vi "Serial_Port_Packet_Read_Write_Test.vi"() -> ()   [LabVIEW 2017]
uses:
  Classes/ADCP.lvclass
panel:
  out "Packet frame ID":u8
  out "Packet node ID":u8
  out "Packet Type":T1(ring)
  out "Checksum Valid ?":bool
  out "Packet_Priority":enum16{"LOW", "HIGH"}(ring)
  out "Raw Packet Out":u8[](array[numeric])
  in  "Raw Packet In":u8[](array[numeric])
  in  "error in (no error)":errorcluster
  in  "Baud rate":u32
  in  "COM Port":refnum<visa-resource-name>
  in  "ADCP in":refnum<class "ADCP.lvclass">
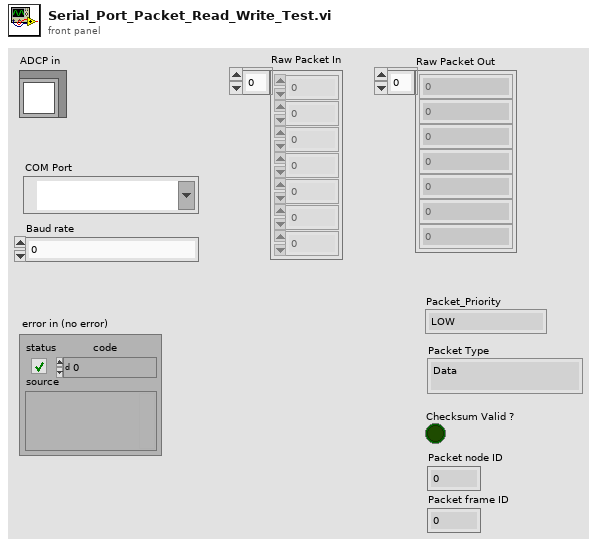
[diagram p1: front panel]
types:
  T1 = enum16{"Data", "Connection Management", "Remote Request", "Error and status", "INVALID"}
  T2 = cluster{"Symbol File Path":path, "Transmit Log File Path":path, "Receive Log File Path":path, "COM Port":refnum<visa-resource-name>, "Baud rate":u32, "Number of retries":u16, "Retry interval (ms)":u16, "Session start time (ms)":u32, "Current time (ms)":u32, "Serialport timeout (ms)":u32}
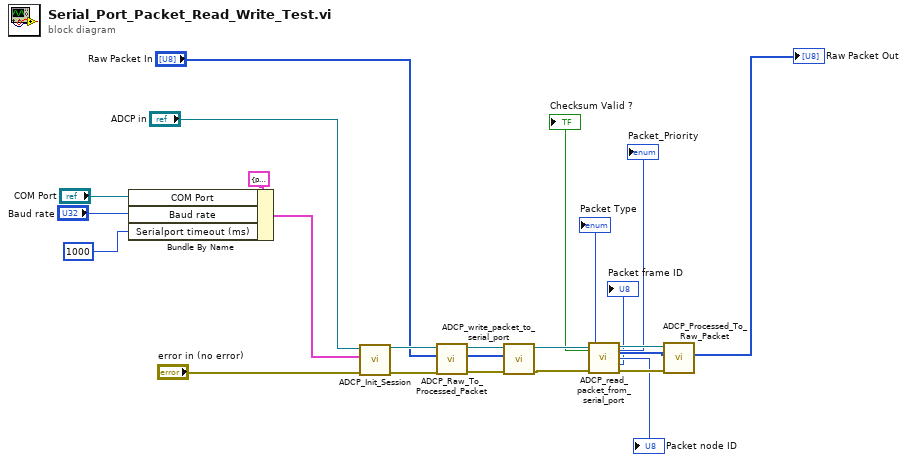
[diagram p0: block diagram]
diagram:
  n1 = Bundle By Name(cluster=T2 {"Symbol File Path"=path "", "Transmit Log File Path"=path "", "Receive Log File Path"=path "", "COM Port"="", "Baud rate"=0, "Number of retries"=0, "Retry interval (ms)"=0, "Session start time (ms)"=0, "Current time (ms)"=0, "Serialport timeout (ms)"=0} ("ADCP Session Parameters"), "COM Port"="COM Port", "Baud rate"="Baud rate", "Serialport timeout (ms)"=u32 1000) -> (w23:T2)
  n2 = call "ADCP_Init_Session.vi"("error in (no error)"="error in (no error)", "ADCP Session Parameters"=w23, "ADCP in"="ADCP in") -> ("error out"=w17:errorcluster, "ADCP out"=w18:refnum<class "ADCP.lvclass">)  [unwired: 7 in]
  n3 = call "ADCP_Raw_To_Processed_Packet.vi"("error in (no error)"=w17, "Raw Packet"="Raw Packet In", "ADCP in"=w18) -> ("error out"=w14:errorcluster, "Processed Packet"=w15:u8[], "ADCP out"=w16:refnum<class "ADCP.lvclass">)  [unwired: 6 in]
  n4 = call "ADCP_write_packet_to_serial_port.vi"("error in (no error)"=w14, "Packet Bytes"=w15, "ADCP In"=w16) -> ("error out"=w11:errorcluster, "ADCP Out"=w12:refnum<class "ADCP.lvclass">)  [unwired: 7 in]
  n5 = call "ADCP_read_packet_from_serial_port.vi"("ADCP In"=w12, "error in (no error)"=w11) -> ("Checksum Valid ?"=→"Checksum Valid ?":bool, "Packet Type"=→"Packet Type":T1, "Packet_Priority"=→"Packet_Priority":enum16{"LOW", "HIGH"}, "ADCP out"=w9:refnum<class "ADCP.lvclass">, "Received Packet"=w8:u8[], "Packet node ID"=→"Packet node ID":u8, "Packet frame ID"=→"Packet frame ID":u8, "error out"=w10:errorcluster)  [unwired: 6 in]
  n6 = call "ADCP_Processed_To_Raw_Packet.vi"("error in (no error)"=w10, "Processed Packet"=w8, "ADCP in"=w9) -> ("Raw Packet"=→"Raw Packet Out":u8[])  [unwired: 6 in, 2 out]
